vi "EvaluateCronExpression.vi"(6 "valid range":cluster{"start":u32, "end":u32}={"start"=0, "end"=59}, 8 "error in (no error)":errorcluster, 10 "expression":string="2, 45, 2-9,* /15", 11 "value":u32) -> (0 "error out":errorcluster, 3 "output":bool)   [LabVIEW 2017, in "CronScheduler.lvlib"]
uses:
  <vilib>/addons/InsightCM/Utilities/CronScheduler/CronScheduler.lvlib
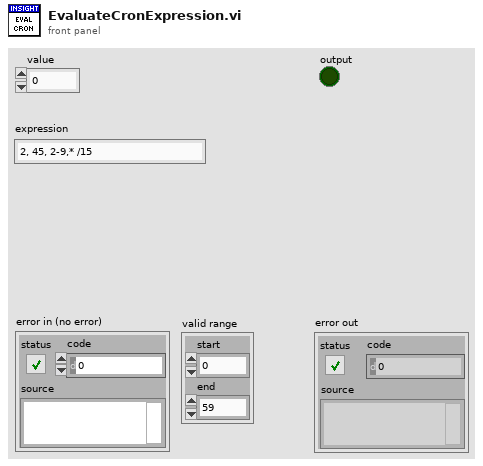
[diagram p1: front panel]
types:
  T1 = typedef "CronScheduler.lvlib/Compare.ctl" = cluster{"compare type":enum16{"any", "number", "range"}, "number":u32, "start":u32, "end":u32}
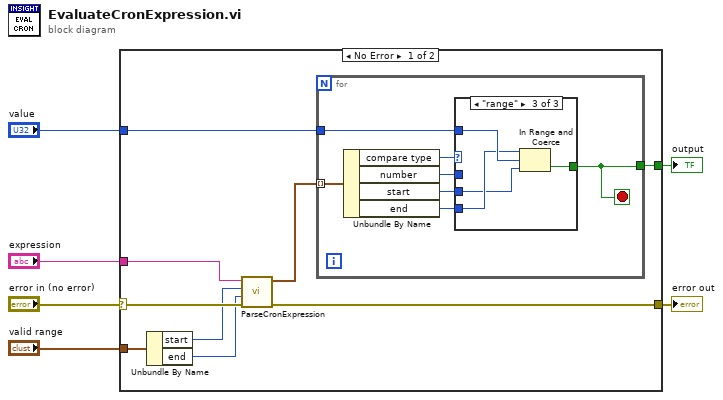
[diagram p0: block diagram]
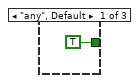
[diagram p2: hidden frame]
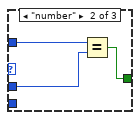
[diagram p3: hidden frame]
diagram:
  n1 = case shown="No Error" "error in (no error)" {
    selector: "error in (no error)" -> [w15 w31]
    tunnel: [w11 w31] -> w5
    tunnel: "value" -> [w12 _]
    tunnel: "expression" -> [w14 _]
    tunnel: [w10 _] -> w2
    tunnel: "valid range" -> [w9 _]
    frame No Error {
      n2 = Unbundle By Name(w9) -> ("start"=w8:u32, "end"=w7:u32)
      n3 = call <vilib>:"ParseCronExpression.vi"("error in (no error)"=w15, "values end"=w7, "values start"=w8, "expression"=w14) -> ("error out"=w11:errorcluster, "comparisons"=w13:T1[])  [unwired: 6 in]
      n4 = for {
        tunnel: w13 -> [w22] mode=indexing
        tunnel: w12 -> [w20]
        tunnel: [w19] -> w10
        stop <- w19 stop-if-true
        n5 = Unbundle By Name(w22) -> ("compare type"=w21:enum16{"any", "number", "range"}, "number"=w18:u32, "start"=w17:u32, "end"=w16:u32)
        n6 = case shown="\"range\"" w21 {
          tunnel: w20 -> [_ w26 w29]
          tunnel: [TRUE w24 w30] -> w19
          tunnel: w18 -> [_ w25 _]
          tunnel: w17 -> [_ _ w27]
          tunnel: w16 -> [_ _ w28]
          frame "any", Default {
          }
          frame "number" {
            n7 = Equal?(x=w26, y=w25) -> (x = y?=w24:bool)
          }
          frame "range" {
            n8 = In Range and Coerce(upper limit=w28, x=w29, lower limit=w27) -> (In Range?=w30:bool)  [unwired: 1 out]
          }
        }
      }
    }
    frame Error {
    }
  }
  "error out" <- w5
  "output" <- w2
